vi "bmi sub vi.vi"(10 "height\n(inches)":dbl, 11 "weight\n(lbs)":dbl) -> (1 "over\nweight":bool, 2 "healthy":bool, 3 "under\nweight":bool, 4 "obese":bool)   [LabVIEW 2018]
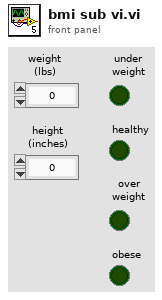
[diagram p1: front panel]
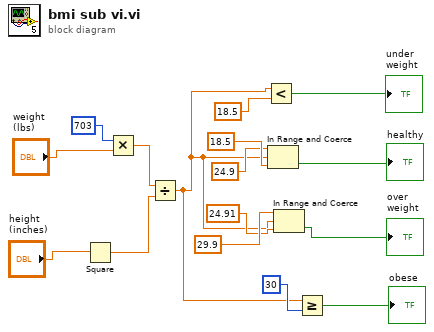
[diagram p0: block diagram]
diagram:
  n1 = Square(x="height\n(inches)") -> (x^2=w5:dbl)
  n2 = Multiply(x=703, y="weight\n(lbs)") -> (x*y=w4:dbl)
  n3 = Divide(x=w4, y=w5) -> (x/y=w11:dbl)
  n4 = Less?(x=w11, y=18.5) -> (x < y?=→"under\nweight":bool)
  n5 = In Range and Coerce(upper limit=24.9, x=w11, lower limit=18.5) -> (In Range?=→"healthy":bool)  [unwired: 1 out]
  n6 = In Range and Coerce(upper limit=29.9, x=w11, lower limit=24.91) -> (In Range?=→"over\nweight":bool)  [unwired: 1 out]
  n7 = Greater Or Equal?(x=w11, y=30) -> (x >= y?=→"obese":bool)
